vi "Launch New Task.vi"(8 "error in (no error)":errorcluster, 9 "Promise":refnum<class "Promise.lvclass">, 10 "Task":refnum<class "Task.lvclass">, 11 "VolatusCoreTask in":refnum<class "VolatusCoreTask.lvclass">) -> (0 "error out":errorcluster, 3 "VolatusCoreTask out":refnum<class "VolatusCoreTask.lvclass">)   [LabVIEW 2020, in "Volatus.lvlib" / "VolatusCoreTask.lvclass"]
uses:
  VolatusCoreTask.lvclass
  C:/dev/lv20CE/relink/lv-volatus/Volatus/Task/Task.lvclass
  Task/Task.lvclass
  lv-promises/Promises/Promise/Promise.lvclass
  TaskEnQrValue/TaskEnQrValue.lvclass/TaskEnQrValue.ctl
  TaskEnQrValue/TaskEnQrValue.lvclass
  C:/dev/lv20CE/relink/lv-promises/Promises/Value/Value.lvclass
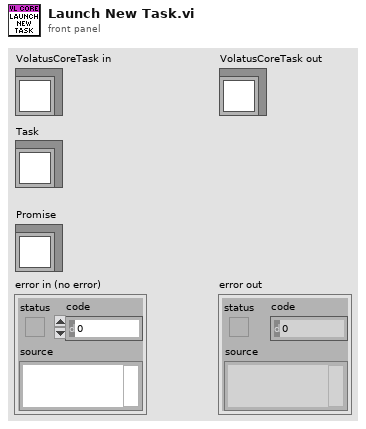
[diagram p1: front panel]
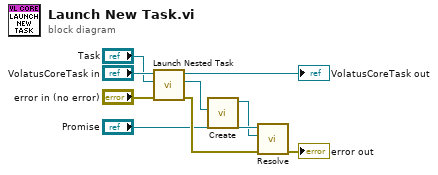
[diagram p0: block diagram]
diagram:
  n1 = call "Launch Nested Task.vi"("error in (no error)"="error in (no error)", "Nested Task"="Task", "Task in"="VolatusCoreTask in") -> ("error out"=w9:errorcluster, "Nested EnQr"=w4:refnum<class "Message Enqueuer.lvclass">, "Task out"=→"VolatusCoreTask out":refnum<class "VolatusCoreTask.lvclass">)  [unwired: 6 in]
  n2 = call "Create.vi"("EnQr"=w4) -> ("TaskEnQrValue out"=w2:refnum<class "TaskEnQrValue.lvclass">)  [unwired: 10 in]
  n3 = call "Resolve.vi"("error in (no error)"=w9, "Result"=w2, "Promise in"="Promise") -> ("error out"=→"error out":errorcluster)  [unwired: 7 in, 1 out]
